vi "updateEnt_hist.vi"() -> ()   [LabVIEW 2012]
uses:
  <vilib>/addons/database/Connection.llb/DB Tools Open Connec (Path).vi
  <vilib>/addons/database/Connection.llb/Conn Execute.vi
  <vilib>/addons/database/Recordset.llb/Rec Fetch Integer Data (R).vi
  <vilib>/addons/database/Recordset.llb/Rec Destroy - Connection.vi
  <vilib>/addons/database/NI_Database_API.lvlib
panel:
  out "error out 2":errorcluster
  in  "Cluster 2":T1 {"Run Site" format="%#_2f"; "Ratio" format="%.3f"}
  in  "End":string="2015/03/20 12:00:00.000"
  in  "Start":string="2015/03/20 08:00:00.000"
  in  "Run Site":i32 format="%.2f"
  in  "Cluster":T1 {"Ratio" format="%.3f"}
  in  "Event":string
  in  "Entity":string
  out "error out":errorcluster
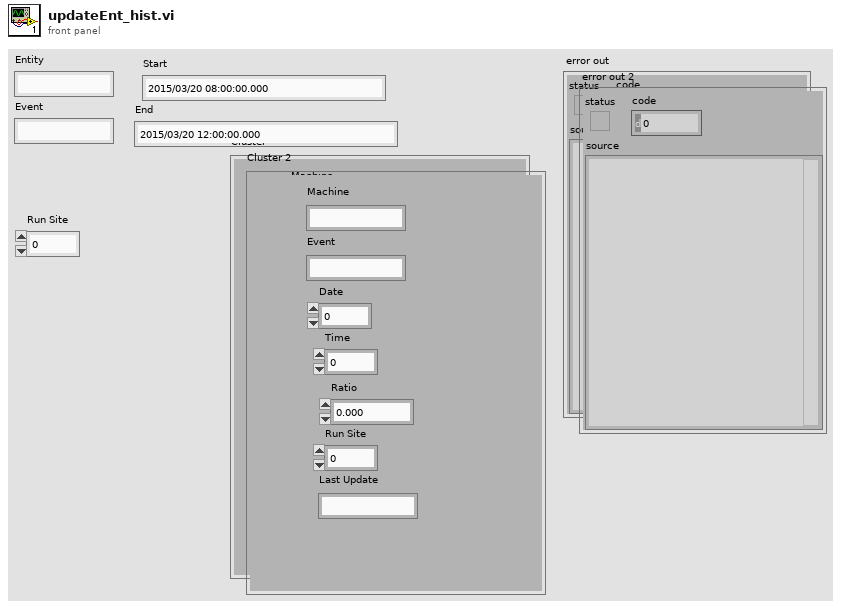
[diagram p1: front panel]
types:
  T1 = cluster{"Machine":string, "Event":string, "Date":dbl, "Time":dbl, "Ratio":dbl, "Run Site":dbl, "Last Update":string}
  T2 = typedef "NI_Database_API.lvlib/Conn ObjectReference.ctl" = refnum<k1>
  T3 = typedef "NI_Database_API.lvlib/Rec ObjectReference.ctl" = refnum<k1>
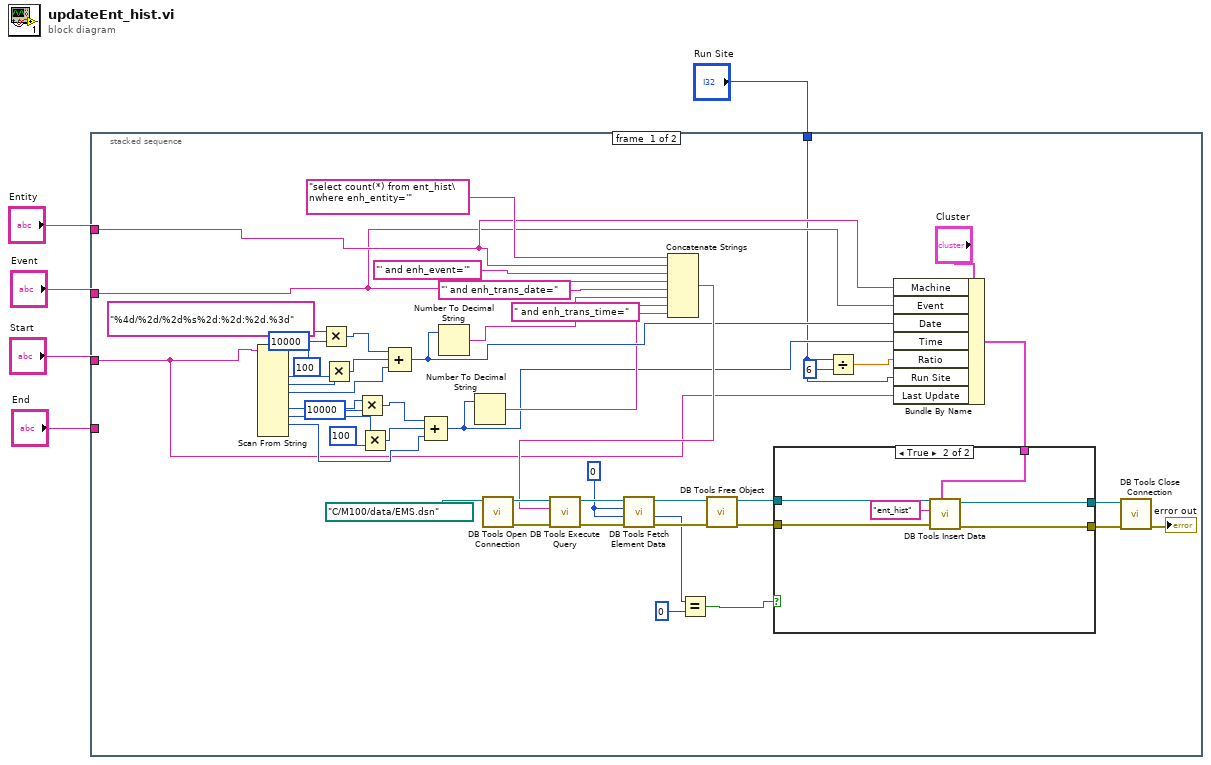
[diagram p0: block diagram]
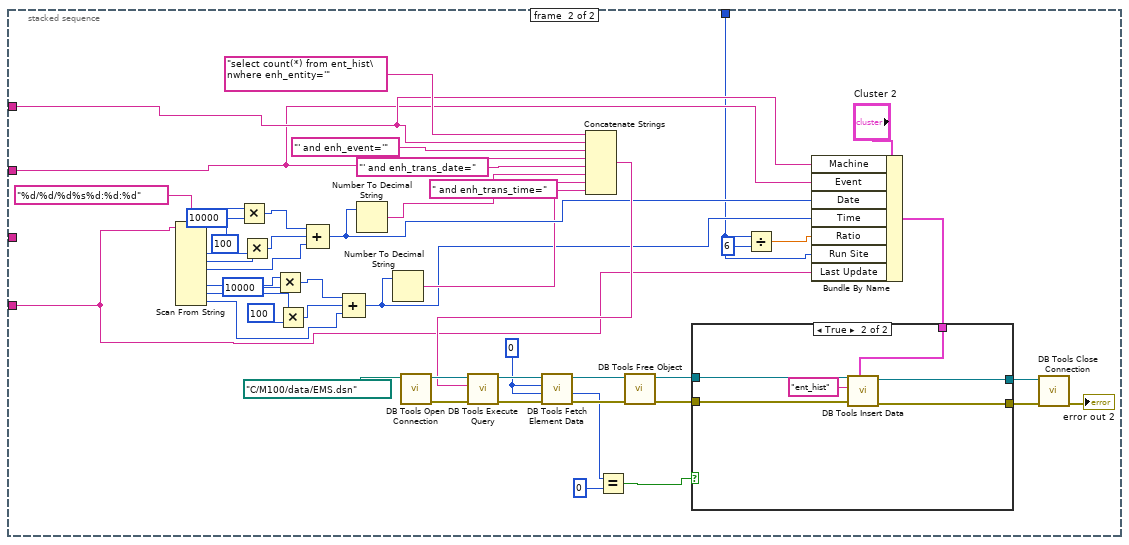
[diagram p3: hidden frame]
diagram:
  n1 = stacked-sequence {
    tunnel: "Entity" -> [w28 w84]
    tunnel: "Event" -> [w27 w83]
    tunnel: "Start" -> [w7 _]
    tunnel: "End" -> [_ w63]
    tunnel: "Run Site" -> [w6 w62]
    frame #0 {
      w41 = 0
      n2 = Scan From String(format string="%4d/%2d/%2d%s%2d:%2d:%2d.%3d", input string=w7) -> (output 1=w25:i32, output 2=w23:i32, output 3=w19:i32, output 5=w12:i32, output 6=w11:i32, output 7=w10:i32)  [unwired: 12 in, 3 out]
      n3 = Multiply(x=w25, y=10000) -> (x*y=w21:i32)
      n4 = Multiply(x=w23, y=100) -> (x*y=w20:i32)
      n5 = Multiply(x=w12, y=10000) -> (x*y=w14:i32)
      n6 = Multiply(x=w11, y=100) -> (x*y=w13:i32)
      n7 = Compound Arithmetic op=ADD(w21, w20, w19) -> (w17:i32)
      n8 = Compound Arithmetic op=ADD(w14, w13, w10) -> (w8:i32)
      n9 = Number To Decimal String(number=w17) -> (decimal integer string=w18:string)  [unwired: 1 in]
      n10 = Number To Decimal String(number=w8) -> (decimal integer string=w9:string)  [unwired: 1 in]
      n11 = call-poly <vilib>:"DB Tools Open Connection.vi"("connection information"=path "C:/M100/data/EMS.dsn") -> ("error out"=w49:errorcluster, "connection reference"=w52:T2)  [unwired: 7 in]
      n12 = Concatenate Strings("select count(*) from ent_hist\nwhere enh_entity='" ("string"), w28, "' and enh_event='" ("string"), w27, "' and enh_trans_date=" ("string"), w18, " and enh_trans_time=" ("string"), w9) -> (w42:string)
      n13 = call-poly <vilib>:"DB Tools Execute Query.vi"("error in (no error)"=w49, "SQL query"=w42, "connection reference"=w52) -> ("error out"=w48:errorcluster, "recordset reference"=w51:T3)  [unwired: 5 in]
      n14 = call-poly <vilib>:"DB Tools Fetch Element Data.vi"("error in (no error)"=w48, "type"=w41, "column index"=w41, "recordset reference"=w51) -> ("error out"=w47:errorcluster, "data"=w39:i32, "recordset reference out"=w50:T3)  [unwired: 3 in]
      n15 = Equal?(x=w39, y=0) -> (x = y?=w37:bool)
      n16 = call-poly <vilib>:"DB Tools Free Object.vi"("error in (no error)"=w47, "recordset reference"=w50) -> ("error out"=w34:errorcluster, "connection reference"=w36:T2)  [unwired: 8 in]
      n17 = Divide(x=w6, y=6) -> (x/y=w30:dbl)
      n18 = Bundle By Name(cluster="Cluster", "Machine"=w28, "Event"=w27, "Date"=w17, "Time"=w8, "Ratio"=w30, "Run Site"=w6, "Last Update"=w7) -> (w29:T1)
      n19 = case shown="True" w37 {
        tunnel: w36 -> [w55 w61]
        tunnel: [w55 w60] -> w35
        tunnel: w34 -> [w54 w59]
        tunnel: [w54 w58] -> w33
        tunnel: w29 -> [_ w57]
        frame False {
        }
        frame True {
          n20 = call <vilib>:"DB Tools Insert Data.vi"("data"=w57, "error in (no error)"=w59, "table"="ent_hist", "connection reference"=w61) -> ("error out"=w58:errorcluster, "connection reference out"=w60:T2)  [unwired: 6 in]
        }
      }
      n21 = call <vilib>:"DB Tools Close Connection.vi"("error in (no error)"=w33, "connection reference"=w35) -> ("error out"=→"error out":errorcluster)  [unwired: 5 in]
    }
    frame #1 {
      w97 = 0
      n22 = Scan From String(format string="%d/%d/%d%s%d:%d:%d", input string=w63) -> (output 1=w81:i32, output 2=w79:i32, output 3=w75:i32, output 5=w68:i32, output 6=w67:i32, output 7=w66:i32)  [unwired: 10 in, 3 out]
      n23 = Multiply(x=w81, y=10000) -> (x*y=w77:i32)
      n24 = Multiply(x=w79, y=100) -> (x*y=w76:i32)
      n25 = Multiply(x=w68, y=10000) -> (x*y=w70:i32)
      n26 = Multiply(x=w67, y=100) -> (x*y=w69:i32)
      n27 = Compound Arithmetic op=ADD(w77, w76, w75) -> (w73:i32)
      n28 = Compound Arithmetic op=ADD(w70, w69, w66) -> (w64:i32)
      n29 = Number To Decimal String(number=w73) -> (decimal integer string=w74:string)  [unwired: 1 in]
      n30 = Number To Decimal String(number=w64) -> (decimal integer string=w65:string)  [unwired: 1 in]
      n31 = call-poly <vilib>:"DB Tools Open Connection.vi"("connection information"=path "C:/M100/data/EMS.dsn") -> ("error out"=w105:errorcluster, "connection reference"=w108:T2)  [unwired: 7 in]
      n32 = Concatenate Strings("select count(*) from ent_hist\nwhere enh_entity='" ("string"), w84, "' and enh_event='" ("string"), w83, "' and enh_trans_date=" ("string"), w74, " and enh_trans_time=" ("string"), w65) -> (w98:string)
      n33 = call-poly <vilib>:"DB Tools Execute Query.vi"("error in (no error)"=w105, "SQL query"=w98, "connection reference"=w108) -> ("error out"=w104:errorcluster, "recordset reference"=w107:T3)  [unwired: 5 in]
      n34 = call-poly <vilib>:"DB Tools Fetch Element Data.vi"("error in (no error)"=w104, "type"=w97, "column index"=w97, "recordset reference"=w107) -> ("error out"=w103:errorcluster, "data"=w95:i32, "recordset reference out"=w106:T3)  [unwired: 3 in]
      n35 = Equal?(x=w95, y=0) -> (x = y?=w93:bool)
      n36 = call-poly <vilib>:"DB Tools Free Object.vi"("error in (no error)"=w103, "recordset reference"=w106) -> ("error out"=w90:errorcluster, "connection reference"=w92:T2)  [unwired: 8 in]
      n37 = Divide(x=w62, y=6) -> (x/y=w86:dbl)
      n38 = Bundle By Name(cluster="Cluster 2", "Machine"=w84, "Event"=w83, "Date"=w73, "Time"=w64, "Ratio"=w86, "Run Site"=w62, "Last Update"=w63) -> (w85:T1)
      n39 = case shown="True" w93 {
        tunnel: w92 -> [w111 w117]
        tunnel: [w111 w116] -> w91
        tunnel: w90 -> [w110 w115]
        tunnel: [w110 w114] -> w89
        tunnel: w85 -> [_ w113]
        frame False {
        }
        frame True {
          n40 = call <vilib>:"DB Tools Insert Data.vi"("data"=w113, "error in (no error)"=w115, "table"="ent_hist", "connection reference"=w117) -> ("error out"=w114:errorcluster, "connection reference out"=w116:T2)  [unwired: 6 in]
        }
      }
      n41 = call <vilib>:"DB Tools Close Connection.vi"("error in (no error)"=w89, "connection reference"=w91) -> ("error out"=→"error out 2":errorcluster)  [unwired: 5 in]
    }
  }
